vi "Final.vi"() -> ()   [LabVIEW 2019]
uses:
  Program Files (x86)/National Instruments/LabVIEW 2019/project/EN1Course-master (12)/EN1Course-master/_Subs/ThingWorx/_TW_Subs/TW_XControl.xctl
panel:
  out "Property (str)":string
  in  "Puzzle Color 5":string(xcontrol)
  in  "Puzzle Color 4":string(xcontrol)
  in  "Puzzle Color 3":string(xcontrol)
  in  "Puzzle Color 2":string(xcontrol)
  in  "Puzzle Color":string(xcontrol)
  in  "Puzzle Color":string(xcontrol)
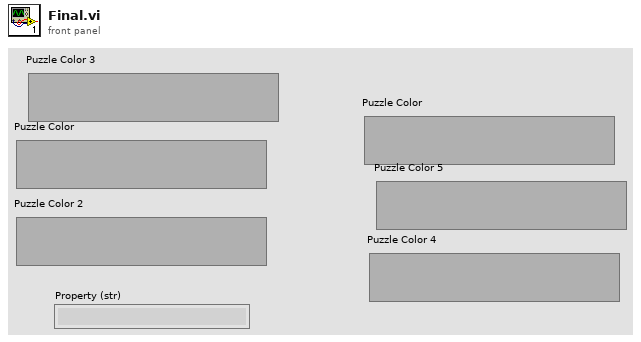
[diagram p1: front panel]
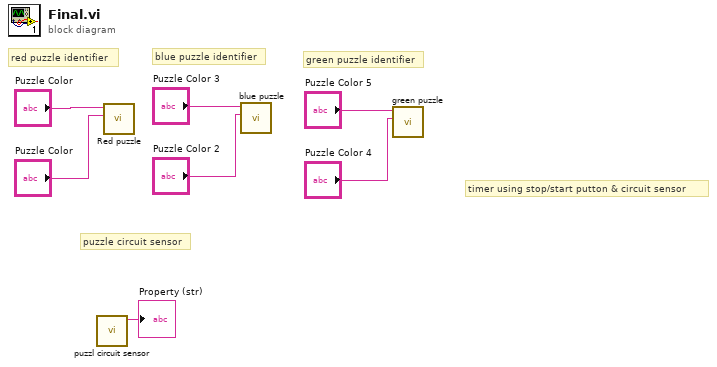
[diagram p0: block diagram]
diagram:
  # "timer using stop/start putton & circuit sensor"
  # "puzzle circuit sensor"
  # "green puzzle identifier"
  # "blue puzzle identifier"
  # "red puzzle identifier"
  n1 = call "puzzl circuit sensor.vi"() -> ("Property (str)"=→"Property (str)":string)  [unwired: 11 in]
  n2 = call "Red puzzle.vi"("Puzzle Color"="Puzzle Color", "Puzzle Color 2"="Puzzle Color") -> ()  [unwired: 10 in]
  n3 = call "blue puzzle.vi"("Puzzle Color in"="Puzzle Color 2", "Puzzle Color 3"="Puzzle Color 3") -> ()  [unwired: 10 in]
  n4 = call "green puzzle.vi"("Puzzle Color 4"="Puzzle Color 4", "Puzzle Color 5"="Puzzle Color 5") -> ()  [unwired: 10 in]
